vi "Reorder 1D Array (EXT).vi"(10 "Sorted Pointers in":i32[](array[numeric]), 11 "Array in":ext[](array[numeric]) format="%.2f") -> (2 "Sorted Pointers out":i32[](array[numeric]), 3 "Sorted Array out":ext[](array[numeric]) format="%.2f")   [LabVIEW 2020]
doc: "This VI reorders a 1D array of any size based on the sorted pointers you specify.\n\n<B>THIS VI IS DEPRICATED</B>. Please use \"Reorder Array2\" (or newer version), available as \"Reorder Array\" from the Functions palette."
panel:
  # "THIS VI IS DEPRICATED.  Please use \"Reorder Array2\" (or newer version), available as \"Reorder Array\" from the Functions palette."
  # "Reorder 1D Array\n\nThis VI reorders a 1D array of any size based on the sorted pointers you specify.\n\nPlease visit http://www.OpenG.org to learn about the\nOpen Source LabVIEW software movement.\n\nNOTICE -- YOU MUST LEAVE THIS NOTICE IN PLACE.  PER THE TERMS OF THE LICENSE BELOW, YOU MAY SUBLICENSE THIS SOFTWARE \nIN ANY WAY THAT DOES NOT CONFLICT WITH THIS LICENSE.\n\n### BSD License (http://www.opensource.org/licenses/bsd-license.php) Begin ###\n \nCopyright (c) 2002, Jim Kring <jim@jimkring.com>\nCopyright (c) 2002, Cal-Bay Systems, Inc. <info@calbay.com>\nCopyright (c) 2005, MKS Instruments, Inc., author: Doug Femec<doug_femec@mksinst.com>, IM dafemec\n\nAll rights reserved.\n\nRedistribution and use in source and binary forms, with or without modification, are permitted provided that the following conditions are met:\n\n    * Redistributions of source code must retain the above copyright notice, this list of conditions and the following disclaimer.\n    * Redistributions in binary form must reproduce the above copyright notice, this list of conditions and the following disclaimer in the \n       documentation and/or other materials provided with the distribution.\n    * Neither the name of SciWare, James Kring, Inc., nor the names of its contributors may be used to endorse or promote products derived \n       from this software without specific prior written permission.\n\nTHIS SOFTWARE IS PROVIDED BY THE COPYRIGHT HOLDERS AND CONTRIBUTORS \"AS IS\" AND ANY EXPRESS OR IMPLIED WARRANTIES, \nINCLUDING, BUT NOT LIMITED TO, THE IMPLIED WARRANTIES OF MERCHANTABILITY AND FITNESS FOR A PARTICULAR PURPOSE ARE \nDISCLAIMED. IN NO EVENT SHALL THE COPYRIGHT OWNER OR CONTRIBUTORS BE LIABLE FOR ANY DIRECT, INDIRECT, INCIDENTAL,\n SPECIAL, EXEMPLARY, OR CONSEQUENTIAL DAMAGES (INCLUDING, BUT NOT LIMITED TO, PROCUREMENT OF SUBSTITUTE GOODS OR \nSERVICES; LOSS OF USE, DATA, OR PROFITS; OR BUSINESS INTERRUPTION) HOWEVER CAUSED AND ON ANY THEORY OF LIABILITY, \nWHETHER IN CONTRACT, STRICT LIABILITY, OR TORT (INCLUDING NEGLIGENCE OR OTHERWISE) ARISING IN ANY WAY OUT OF THE USE \nOF THIS SOFTWARE, EVEN IF ADVISED OF THE POSSIBILITY OF SUCH DAMAGE.\n\n### BSD License End ###"
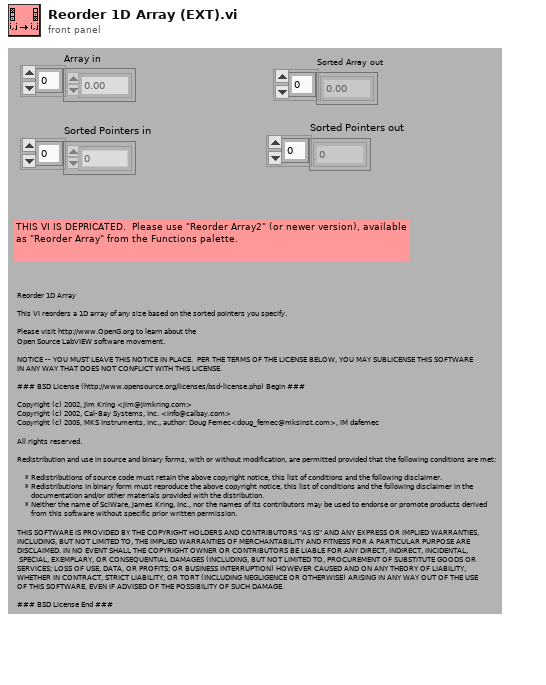
[diagram p1: front panel]
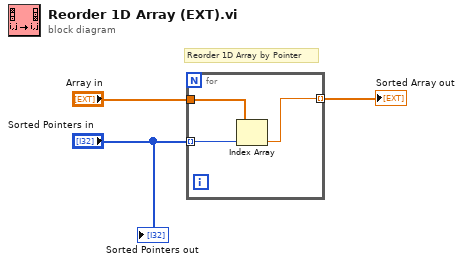
[diagram p0: block diagram]
diagram:
  # "Reorder 1D Array by Pointer"
  n1 = for {
    tunnel: "Array in" -> [w6]
    tunnel: [w5] -> w2 mode=indexing
    tunnel: "Sorted Pointers in" -> [w4] mode=indexing
    n2 = Index Array(array=w6, index=w4) -> (element=w5:ext)
  }
  "Sorted Array out" <- w2
  "Sorted Pointers out" <- "Sorted Pointers in"
